vi "MathOptim-Fit Sigmoid.vi"(0 "Y":dbl[](array[numeric]), 5 "X":dbl[](array[numeric]), 11 "error in (no error)":errorcluster) -> (4 "best nonlinear fit":dbl[](array[numeric]), 6 "best fit parameters":dbl[](array[numeric]), 8 "SSE":dbl, 10 "adjusted R2":dbl, 14 "summary":string, 15 "error out":errorcluster)   [LabVIEW 2020]
uses:
  <vilib>/gmath/NumericalOptimization/Nonlinear Curve Fit LM.vi
  <vilib>/gmath/NI_Gmath.lvlib
panel:
  out "R2":dbl
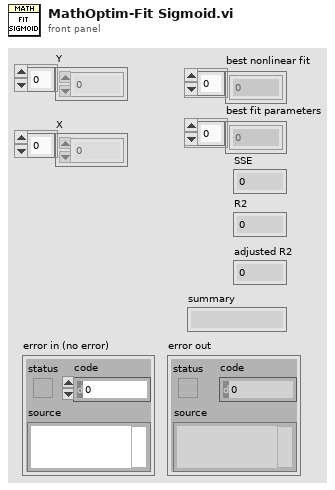
[diagram p1: front panel]
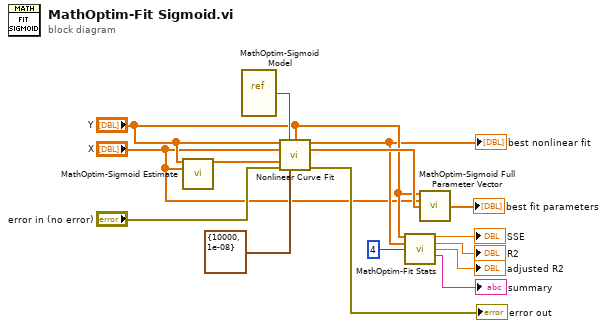
[diagram p0: block diagram]
diagram:
  n1 = call "MathOptim-Sigmoid Estimate.vi"("Y"="Y", "X"="X") -> ("Initial guess"=w12:dbl[])  [unwired: 13 in]
  n2 = vi-ref "MathOptim-Sigmoid Model.vi"() -> (w15:refnum<vi>)
  n3 = call-poly <vilib>:"Nonlinear Curve Fit.vi"("Y"="Y", "f(x,a)"=w15, "data"="Y", "X"="X", "initial parameters"=w12, "error in (no error)"="error in (no error)", "termination"=cluster{"max iteration":i32, "tolerance":dbl} {"max iteration"=10000, "tolerance"=1e-08}) -> ("best nonlinear fit"=w3:dbl[], "best fit parameters"=w5:dbl[], "error out"=→"error out":errorcluster)  [unwired: 3 in, 3 out]
  "best nonlinear fit" <- w3
  n4 = call "MathOptim-Fit Stats.vi"("Y"="Y", "Yfit"=w3, "Num params"=4) -> ("SSE"=→"SSE":dbl, "R2"=→"R2":dbl, "adjusted R2"=→"adjusted R2":dbl, "summary"=→"summary":string)  [unwired: 9 in]
  n5 = call "MathOptim-Sigmoid Full Parameter Vector.vi"("Y"="Y", "X"="X", "a"=w5) -> ("Parameters"=→"best fit parameters":dbl[])  [unwired: 12 in]
